vi "Send Output.vi"(8 "error in":errorcluster, 11 "89XX in":refnum<class "89XX.lvclass">) -> (0 "error out":errorcluster, 3 "89XX out":refnum<class "89XX.lvclass">)   [LabVIEW 2019, in "89XX.lvlib" / "89XX.lvclass"]
uses:
  Library/89XX.lvclass
  C:/Users/Public/Documents/Development/builds/Instruments/PowerSupply.lvlibp/Library/PowerSupply.lvclass
  Library/89XX.lvclass/89XX.ctl
  Accessors/Read Local Resource.vi
  <instrlib>/Keysight N8900 Series/Keysight N8900 Series.lvlib
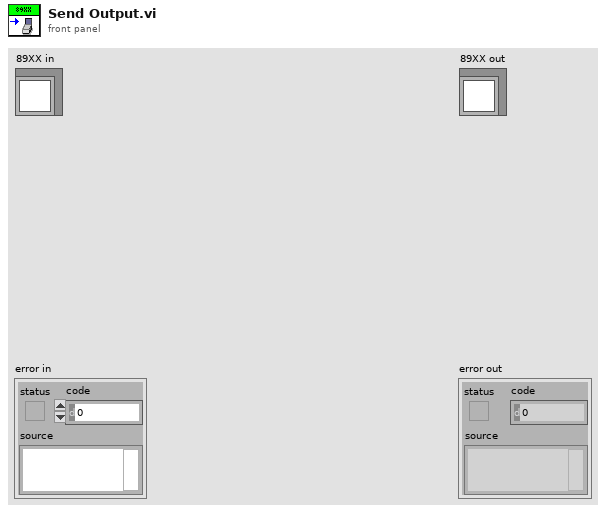
[diagram p1: front panel]
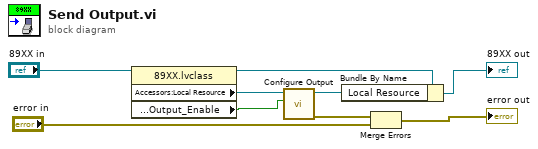
[diagram p0: block diagram]
diagram:
  n1 = property class="89XX.lvclass"(reference="89XX in") -> (reference out=w8:refnum<class "89XX.lvclass">, "Accessors:Local Resource"=w4:refnum<visa-resource-name>, "Accessors:Setting:Output_Enable"=w3:bool)  [unwired: 1 in, 1 out]
  n2 = call <instrlib>:"Configure Output.vi"("Enable Output (F: Disable)"=w3, "VISA resource name"=w4) -> ("error out"=w6:errorcluster, "VISA resource name out"=w5:refnum<visa-resource-name>)  [unwired: 8 in]
  n3 = Bundle By Name(cluster=w8, "Local Resource"=w5) -> (→"89XX out":refnum<class "89XX.lvclass">)
  n4 = Merge Errors(w6, "error in") -> (→"error out":errorcluster)
